vi "update tree control.vi"(8 "error in":errorcluster, 10 "tree reference":refnum<vi>, 11 "glyph manager in":T1) -> (0 "error out":errorcluster, 3 "glyph manager out":T1)   [LabVIEW 2013, in "glyph manager.lvlib"]
uses:
  glyph manager.lvlib
  glyph manager.ctl
  <vilib>/picture/picture.llb/imagedata.ctl
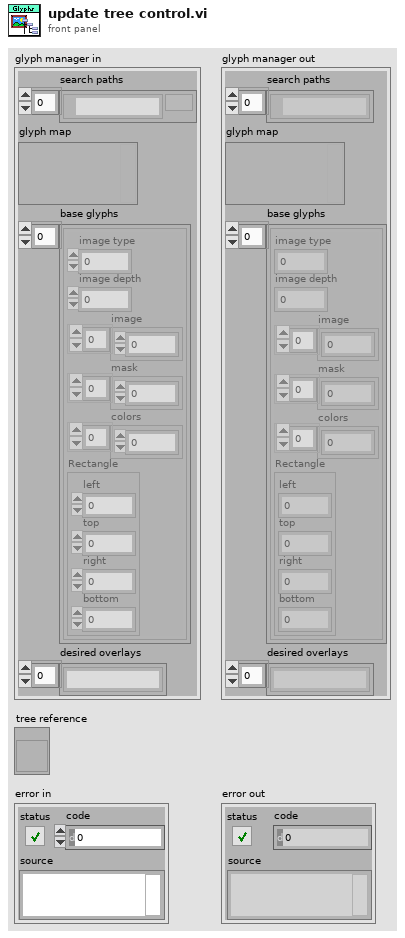
[diagram p1: front panel]
types:
  T1 = typedef "glyph manager.lvlib/glyph manager.ctl" = cluster{"search paths":path[], "glyph map":variant, "base glyphs":T2[], "desired overlays":string[]}
  T2 = typedef "imagedata.ctl" = cluster{"image type":i32, "image depth":i32, "image":u8[], "mask":u8[], "colors":u32[], "Rectangle":cluster{"left":i16, "top":i16, "right":i16, "bottom":i16}}
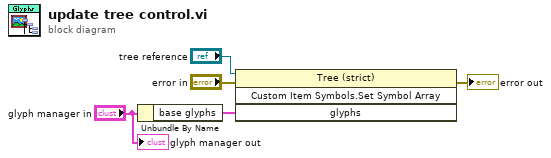
[diagram p0: block diagram]
diagram:
  n1 = Unbundle By Name("glyph manager in") -> ("base glyphs"=w1:T2[])
  n2 = invoke class="Tree (strict)" method="Custom Item Symbols.Set Symbol Array"(reference="tree reference", error in="error in", "glyphs"=w1) -> (error out=→"error out":errorcluster)  [unwired: 1 in, 3 out]
  "glyph manager out" <- "glyph manager in"
